vi "零件加工.vi"() -> ()   [LabVIEW 2011]
panel:
  out "Output":string
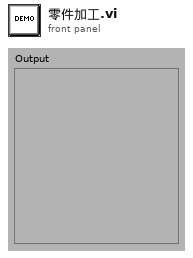
[diagram p1: front panel]
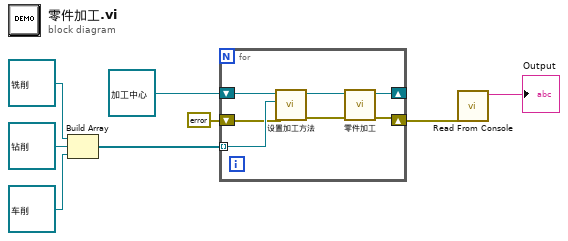
[diagram p0: block diagram]
diagram:
  n1 = Build Array(refnum<class "铣削.lvclass"> refnum ("铣削.lvclass"), refnum<class "钻削.lvclass"> refnum ("钻削.lvclass"), refnum<class "车削.lvclass"> refnum ("车削.lvclass")) -> (w4:refnum<class "加工类（抽象）.lvclass">[])
  n2 = for {
    shift-right: [w12] -> _
    shift-left: refnum<class "加工中心.lvclass"> refnum ("加工中心.lvclass") -> [w15]
    tunnel: w4 -> [w11] mode=indexing
    shift-right: [w10] -> w2
    shift-left: errorcluster {"status"=FALSE, "code"=0, "source"=""} ("error out") -> [w9]
    n3 = call "设置加工方法.vi"("error in (no error)"=w9, "加工类（抽象）.lvclass"=w11, "加工中心 输入"=w15) -> ("error out"=w13:errorcluster, "加工中心 输出"=w14:refnum<class "加工中心.lvclass">)  [unwired: 7 in]
    n4 = call "零件加工.vi"("error in (no error)"=w13, "加工中心 输入"=w14) -> ("error out"=w10:errorcluster, "加工中心 输出"=w12:refnum<class "加工中心.lvclass">)  [unwired: 8 in]
  }
  n5 = call "Read From Console.vi"("error in (no error)"=w2) -> ("Output"=→"Output":string)  [unwired: 9 in, 1 out]
